vi "TempDisplay.vi"(0 "VisaCluster":T2, 7 "Temp_Unit":T1, 11 "error in (no error)":errorcluster) -> (4 "VisaCluster 2":T2, 6 "Answer":string, 8 "Temp_Unit 2":T1, 15 "error out":errorcluster)   [LabVIEW 2014, in "FH 55.lvlib"]
doc: "Dieses VI gibt nur den aktuellen Temperaturwert zurück wenn Celsius oder Fahrenheit übergeben wird.\n\nThis VI returns only the current temperature where Celsius and Fahrenheit is inputted."
uses:
  FH 55.lvlib
  TypeDef/VisaCluster.ctl
  TypeDef/Temp_Unit.ctl
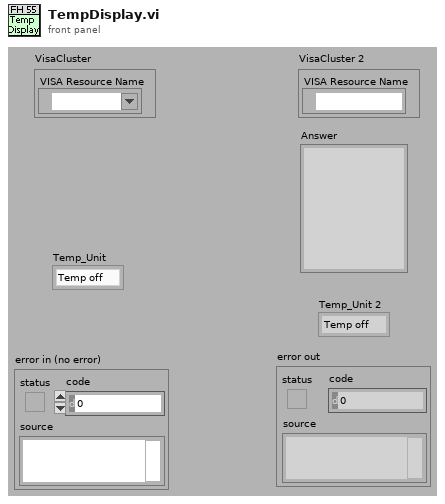
[diagram p1: front panel]
types:
  T1 = typedef "FH 55.lvlib/Temp_Unit.ctl" = enum16{"Temp off", "Celsius", "Fahrenheit"}
  T2 = typedef "FH 55.lvlib/VisaCluster.ctl" = cluster{"VISA Resource Name":refnum<visa-resource-name>}
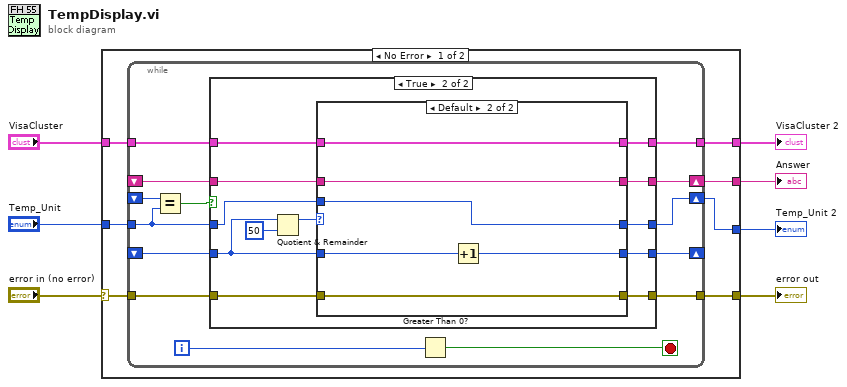
[diagram p0: block diagram]
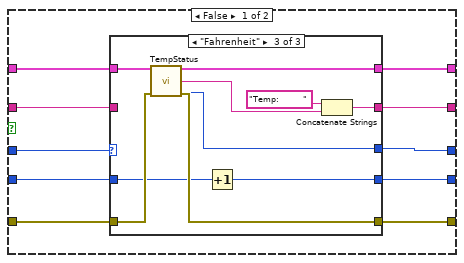
[diagram p2: hidden frame]
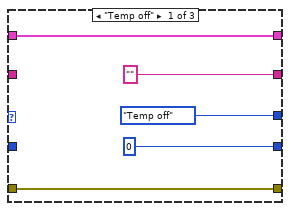
[diagram p3: hidden frame]
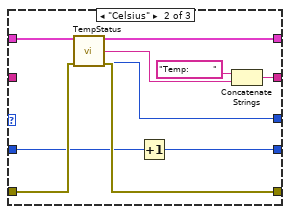
[diagram p4: hidden frame]
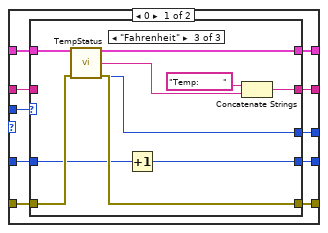
[diagram p5: hidden frame]
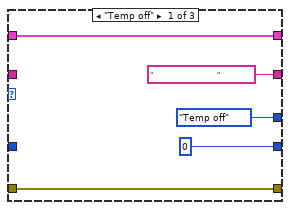
[diagram p6: hidden frame]
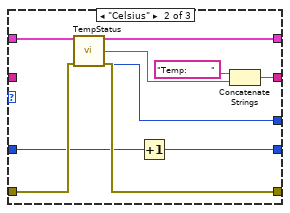
[diagram p7: hidden frame]
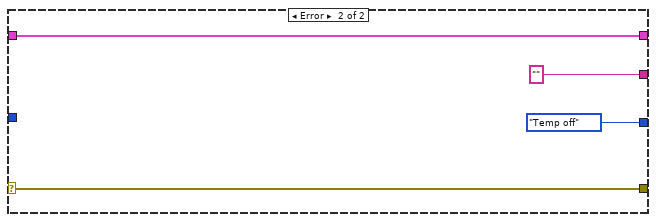
[diagram p8: hidden frame]
diagram:
  n1 = case shown="No Error" "error in (no error)" {
    selector: "error in (no error)" -> [w11 w119]
    tunnel: [w8 Temp_Unit."Temp off" ("Temp_Unit")] -> w1
    tunnel: [w14 "" ("Answer")] -> w7
    tunnel: "VisaCluster" -> [w13 w120]
    tunnel: "Temp_Unit" -> [w12 _]
    tunnel: [w9 w120] -> w4
    tunnel: [w10 w119] -> w3
    frame No Error {
      n2 = while {
        tunnel: w13 -> [w27]
        tunnel: w12 -> [w16]
        tunnel: w11 -> [w26]
        tunnel: [w25] -> w10
        tunnel: [w24] -> w9
        shift-right: [w20] -> _
        shift-left: _ -> [w18]
        shift-right: [w28] -> w14
        shift-left: _ -> [w19]
        shift-right: [w23] -> w8
        shift-left: _ -> [w17]
        i -> [w22]
        stop <- w21 stop-if-true
        n3 = Equal?(x=w17, y=w16) -> (x = y?=w15:bool)
        n4 = case shown="True" w15 {
          tunnel: [w32 w75] -> w28
          tunnel: w27 -> [w38 w74]
          tunnel: w16 -> [w36 w73]
          tunnel: w26 -> [w34 w72]
          tunnel: [w29 w71] -> w25
          tunnel: [w33 w70] -> w24
          tunnel: [w31 w69] -> w23
          tunnel: [w30 w68] -> w20
          tunnel: w19 -> [w37 w67]
          tunnel: w18 -> [w35 w66]
          frame False {
            n5 = case shown="\"Fahrenheit\"" w36 {
              tunnel: w38 -> [w41 w53 w63]
              tunnel: ["" w48 w58] -> w32
              tunnel: w34 -> [w42 w52 w56]
              tunnel: [w42 w51 w62] -> w29
              tunnel: [w41 w50 w61] -> w33
              tunnel: [Temp_Unit."Temp off" ("Temp_Unit") w49 w60] -> w31
              tunnel: w35 -> [_ w45 w55]
              tunnel: [i64 0 w44 w54] -> w30
              tunnel: w37 -> [_ _ _]
              frame "Temp off" {
              }
              frame "Celsius" {
                n6 = call "TempStatus.vi"("VisaCluster"=w53, "error in (no error)"=w52) -> ("VisaCluster"=w50:T2, "Answer"=w46:string, "Temp_Unit"=w49:T1, "error out"=w51:errorcluster)  [unwired: 10 in]
                n7 = Increment(x=w45) -> (x+1=w44:i64)
                n8 = Concatenate Strings("Temp:        ", w46) -> (w48:string)
              }
              frame "Fahrenheit" {
                n9 = call "TempStatus.vi"("VisaCluster"=w63, "error in (no error)"=w56) -> ("VisaCluster"=w61:T2, "Answer"=w57:string, "Temp_Unit"=w60:T1, "error out"=w62:errorcluster)  [unwired: 10 in]
                n10 = Increment(x=w55) -> (x+1=w54:i64)
                n11 = Concatenate Strings("Temp:        ", w57) -> (w58:string)
              }
            }
          }
          frame True {
            n12 = Quotient & Remainder(x=w66, y=i64 50) -> (x-y*floor(x/y)=w64:i64)  [unwired: 1 out]
            n13 = case shown="Default" w64 {
              tunnel: [w85 w116] -> w75
              tunnel: w74 -> [w84 w111]
              tunnel: w73 -> [w83 w115]
              tunnel: w72 -> [w82 w112]
              tunnel: [w81 w112] -> w71
              tunnel: [w80 w111] -> w70
              tunnel: [w79 w115] -> w69
              tunnel: w66 -> [w78 w114]
              tunnel: [w77 w113] -> w68
              tunnel: w67 -> [w76 w116]
              frame 0 {
                n14 = case shown="\"Fahrenheit\"" w83 {
                  tunnel: w84 -> [w88 w100 w110]
                  tunnel: ["                                " w95 w105] -> w85
                  tunnel: w82 -> [w89 w99 w103]
                  tunnel: [w89 w98 w109] -> w81
                  tunnel: [w88 w97 w108] -> w80
                  tunnel: [Temp_Unit."Temp off" ("Temp_Unit") w96 w107] -> w79
                  tunnel: w78 -> [_ w92 w102]
                  tunnel: [i64 0 w91 w101] -> w77
                  tunnel: w76 -> [_ _ _]
                  frame "Temp off" {
                  }
                  frame "Celsius" {
                    n15 = call "TempStatus.vi"("VisaCluster"=w100, "error in (no error)"=w99) -> ("VisaCluster"=w97:T2, "Answer"=w93:string, "Temp_Unit"=w96:T1, "error out"=w98:errorcluster)  [unwired: 10 in]
                    n16 = Increment(x=w92) -> (x+1=w91:i64)
                    n17 = Concatenate Strings("Temp:        ", w93) -> (w95:string)
                  }
                  frame "Fahrenheit" {
                    n18 = call "TempStatus.vi"("VisaCluster"=w110, "error in (no error)"=w103) -> ("VisaCluster"=w108:T2, "Answer"=w104:string, "Temp_Unit"=w107:T1, "error out"=w109:errorcluster)  [unwired: 10 in]
                    n19 = Increment(x=w102) -> (x+1=w101:i64)
                    n20 = Concatenate Strings("Temp:        ", w104) -> (w105:string)
                  }
                }
              }
              frame Default {
                n21 = Increment(x=w114) -> (x+1=w113:i64)
              }
            }
          }
        }
        n22 = Greater Than 0?(x=w22) -> (x > 0?=w21:bool)
      }
    }
    frame Error {
    }
  }
  "Answer" <- w7
  "error out" <- w3
  "VisaCluster 2" <- w4
  "Temp_Unit 2" <- w1
